vi "Eurotherm - VISA Serial - Close Session.vi"(0 "VISA resource name":refnum<visa-resource-name>, 11 "error in (no error)":errorcluster) -> (4 "dup VISA resource name":refnum<visa-resource-name>, 15 "error out":errorcluster)   [LabVIEW 2011]
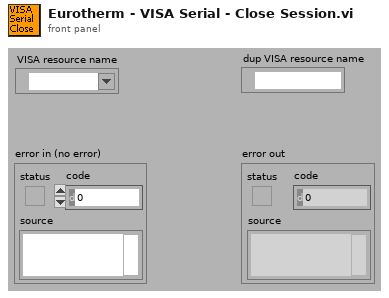
[diagram p1: front panel]
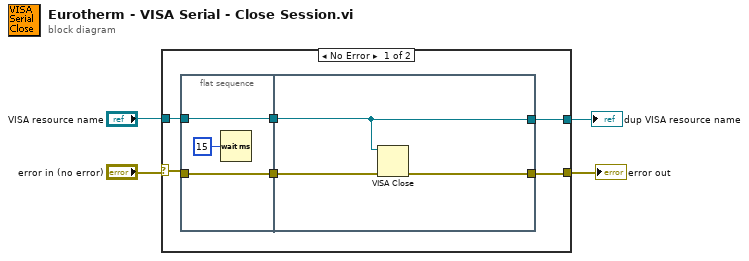
[diagram p0: block diagram]
diagram:
  n1 = case shown="No Error" "error in (no error)" {
    selector: "error in (no error)" -> [w9 w18]
    tunnel: [w10 w18] -> w3
    tunnel: "VISA resource name" -> [w8 w17]
    tunnel: [w5 w17] -> w1
    frame No Error {
      n2 = flat-sequence {
        tunnel: w9 -> [w12]
        tunnel: [w12] -> w7
        tunnel: w8 -> [w11]
        tunnel: [w11] -> w6
        tunnel: [w16] -> w10
        tunnel: w7 -> [w15]
        tunnel: w6 -> [w14]
        tunnel: [w14] -> w5
        frame #0 {
          n3 = Wait (ms)(milliseconds to wait=u32 15) -> ()  [unwired: 1 out]
        }
        frame #1 {
          n4 = VISA Close(VISA resource name=w14, error in (no error)=w15) -> (error out=w16:errorcluster)
        }
      }
    }
    frame Error {
    }
  }
  "error out" <- w3
  "dup VISA resource name" <- w1
